vi "Read Audio Data.vi"(8 "error in (no error)":errorcluster, 10 "Frames":u64, 11 "Channel in":refnum<data-value>) -> (0 "error out":errorcluster, 2 "Audio Data":sgl[][](array[numeric]), 3 "Channel out":refnum<data-value>)   [LabVIEW 2020, in "G-Audio.lvlib" / "Channel.lvclass"]
uses:
  Channel.lvclass
  Channel.lvclass/Channel.ctl
  Channel State.ctl
  <vilib>/Analysis/1siggen.llb/Ramp Pattern by Samples.vi
  <vilib>/Analysis/NI_AALBase.lvlib
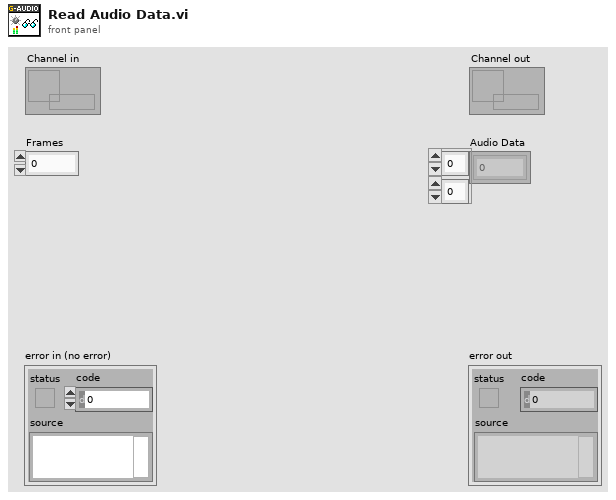
[diagram p1: front panel]
types:
  T1 = typedef "G-Audio.lvlib/Channel.lvclass/Channel State.ctl" = enum16{"Empty", "Loading", "Stopped", "Paused", "Playing", "Retrigger"}
  T2 = typedef "G-Audio.lvlib/Mixer.lvclass/Mixer Audio Data Type.ctl" = i16[][]
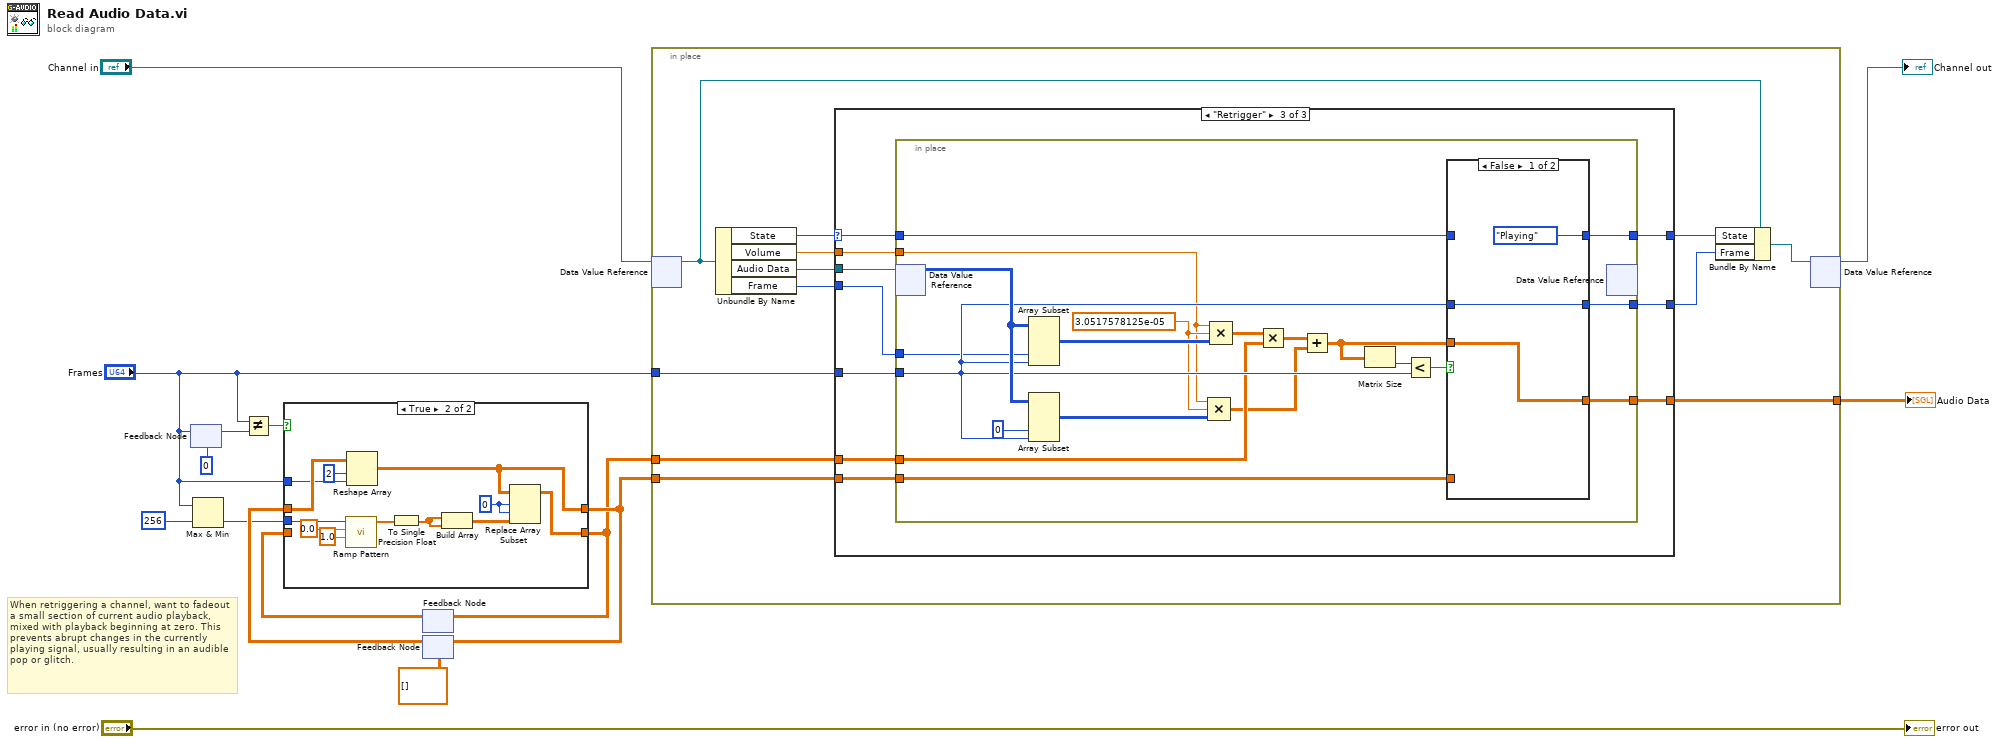
[diagram p0: block diagram]
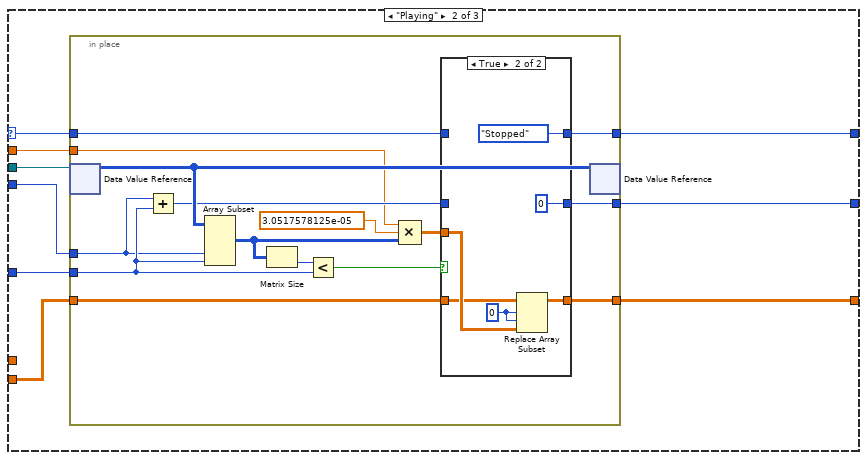
[diagram p3: hidden frame]
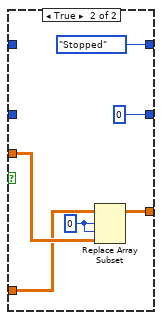
[diagram p5: hidden frame]
diagram:
  # "When retriggering a channel, want to fadeout a small section of current audio playback, mixed with playback beginning at zero. This prevents abrupt changes in the currently playing signal, usually resulting in an audible pop or glitch."
  n1 = feedback #1(u64 0 ("Frames")) -> (w14:u64)
  n2 = feedback-in #1("Frames") -> ()
  n3 = Max & Min(x="Frames", y=u64 256) -> (min(x,y)=w3:u64)  [unwired: 1 out]
  n4 = Not Equal?(x="Frames", y=w14) -> (x != y?=w13:bool)
  n5 = feedback #2() -> (w8:sgl[][])  [unwired: 1 in]
  n6 = feedback #3(sgl[][] [] ("Audio Data Type")) -> (w12:sgl[][])
  n7 = case shown="True" w13 {
    tunnel: "Frames" -> [_ w27]
    tunnel: [w17 w21] -> w11
    tunnel: w12 -> [w17 w29]
    tunnel: [w16 w18] -> w7
    tunnel: w8 -> [w16 _]
    tunnel: w3 -> [_ w22]
    frame False {
    }
    frame True {
      w20 = 0 ("index (row)")
      n8 = call-poly <vilib>:"Ramp Pattern.vi"("start"=1.0, "end"=0.0, "samples"=w22) -> ("Ramp Pattern"=w26:dbl[])  [unwired: 7 in, 1 out]
      n9 = Reshape Array(w29, u64 2 ("dimension size"), w27) -> (w21:sgl[][])
      n10 = To Single Precision Float(number=w26) -> (single precision float=w23:sgl[])
      n11 = Build Array(w23, w23) -> (w19:sgl[][])
      n12 = Replace Array Subset(array=w21, new element=w19, index (row)=w20, index (col)=w20) -> (w18:sgl[][])
    }
  }
  n13 = feedback-in #2(w7) -> ()
  n14 = feedback-in #3(w11) -> ()
  n15 = in-place {
    in-place-border: "Frames" -> [w41]
    in-place-border: [w40] -> w6
    in-place-border: w11 -> [w39]
    in-place-border: w7 -> [w38]
    n16 = in-place-dvr #4("Channel in") -> (w37:refnum<class "Channel.lvclass">)  [unwired: 1 out]
    n17 = Unbundle By Name(w37) -> ("State"=w32:T1, "Volume"=w33:sgl, "Audio Data"=w34:refnum<data-value>, "Frame"=w35:u64)
    n18 = case shown="\"Retrigger\"" w32 {
      selector: w32 -> [w44 w49 w83]
      tunnel: w41 -> [_ w53 w87]
      tunnel: w34 -> [_ w52 w86]
      tunnel: w35 -> [w42 w46 w79]
      tunnel: [w43 w51 w85] -> w40
      tunnel: [w44 w48 w82] -> w31
      tunnel: w39 -> [w43 w50 w84]
      tunnel: w38 -> [_ _ w81]
      tunnel: w33 -> [_ w47 w80]
      tunnel: [w42 w45 w78] -> w30
      frame Default {
      }
      frame "Playing" {
        n19 = in-place {
          in-place-border: w53 -> [w66]
          in-place-border: [w64] -> w51
          in-place-border: w50 -> [w63]
          in-place-border: w49 -> [w61]
          in-place-border: [w60] -> w48
          in-place-border: w47 -> [w56]
          in-place-border: w46 -> [w55]
          in-place-border: [w54] -> w45
          n20 = in-place-dvr #5(w52) -> (w68:T2)  [unwired: 1 out]
          n21 = Add(x=w55, y=w66) -> (x+y=w62:u64)
          n22 = Array Subset(array=w68, index (col)=w55, length (col)=w66) -> (w58:T2)  [unwired: 2 in]
          n23 = Matrix Size(0:w58) -> (2:w67:i32)  [unwired: 1 out]
          n24 = Less?(x=w67, y=w66) -> (x < y?=w65:bool)
          n25 = Compound Arithmetic op=MULTIPLY(w56, sgl 3.0517578e-05, w58) -> (w57:sgl[][])
          n26 = case shown="True" w65 {
            tunnel: [w71 w75] -> w64
            tunnel: w57 -> [w71 w77]
            tunnel: w63 -> [_ w76]
            tunnel: w62 -> [w70 _]
            tunnel: [w70 u64 0] -> w54
            tunnel: w61 -> [w69 _]
            tunnel: [w69 Channel_State."Stopped" ("State")] -> w60
            frame False {
            }
            frame True {
              w74 = 0 ("index (row)")
              n27 = Replace Array Subset(array=w76, new element=w77, index (row)=w74, index (col)=w74) -> (w75:sgl[][])
            }
          }
          n28 = in-place-dvr #5(w68) -> ()  [unwired: 2 out]
        }
      }
      frame "Retrigger" {
        n29 = in-place {
          in-place-border: w87 -> [w100]
          in-place-border: [w105] -> w85
          in-place-border: w84 -> [w104]
          in-place-border: w83 -> [w103]
          in-place-border: [w102] -> w82
          in-place-border: w81 -> [w95]
          in-place-border: w80 -> [w90]
          in-place-border: w79 -> [w89]
          in-place-border: [w88] -> w78
          w91 = sgl 3.0517578e-05
          n30 = in-place-dvr #6(w86) -> (w101:T2)  [unwired: 1 out]
          n31 = Array Subset(array=w101, index (col)=w89, length (col)=w100) -> (w98:T2)  [unwired: 2 in]
          n32 = Array Subset(array=w101, index (col)=0 ("index"), length (col)=w100) -> (w97:T2)  [unwired: 2 in]
          n33 = Compound Arithmetic op=MULTIPLY(w90, w91, w97) -> (w93:sgl[][])
          n34 = Compound Arithmetic op=MULTIPLY(w90, w91, w98) -> (w96:sgl[][])
          n35 = Multiply(x=w96, y=w95) -> (x*y=w94:sgl[][])
          n36 = Add(x=w94, y=w93) -> (x+y=w92:sgl[][])
          n37 = Matrix Size(0:w92) -> (2:w107:i32)  [unwired: 1 out]
          n38 = Less?(x=w107, y=w100) -> (x < y?=w106:bool)
          n39 = case shown="False" w106 {
            tunnel: [w110 w114] -> w105
            tunnel: w92 -> [w110 w116]
            tunnel: w104 -> [_ w115]
            tunnel: w100 -> [w109 _]
            tunnel: [w109 u64 0] -> w88
            tunnel: w103 -> [_ _]
            tunnel: [Channel_State."Playing" ("State") Channel_State."Stopped" ("State")] -> w102
            frame False {
            }
            frame True {
              w113 = 0 ("index (row)")
              n40 = Replace Array Subset(array=w115, new element=w116, index (row)=w113, index (col)=w113) -> (w114:sgl[][])
            }
          }
          n41 = in-place-dvr #6() -> ()  [unwired: 1 in, 2 out]
        }
      }
    }
    n42 = Bundle By Name(cluster=w37, "State"=w31, "Frame"=w30) -> (w36:refnum<class "Channel.lvclass">)
    n43 = in-place-dvr #4(w36) -> (→"Channel out":refnum<data-value>)  [unwired: 1 out]
  }
  "Audio Data" <- w6
  "error out" <- "error in (no error)"
